vi "Abstract MVA Application (Template).vi"   [LabVIEW 2017]
uses:
  Framework/IModel/IModel/IModel.lvclass
  Framework/IViewable/IViewable/IViewable.lvclass
  Framework/IViewModel/IViewModel/IViewModel.lvclass
  C:/Git/mva-framework/Source/Framework/IViewManager/IViewManager/IViewManager.lvclass
  C:/Program Files (x86)/National Instruments/LabVIEW 2017/vi.lib/ActorFramework/Actor/Actor.lvclass
  Framework/Mediator/Mediator/Mediator.lvclass
  C:/Git/mva-framework/Source/Framework/IMediator/IMediator/IMediator.lvclass
  Framework/Mediator/MediatorBusMonitor/MediatorBusMonitor.lvclass
  C:/Git/mva-framework/Source/Framework/IMediator/IMediatorBusMonitor/MediatorBusMonitor/IMediatorBusMonitor.lvclass
  <vilib>/ActorFramework/Message Enqueuer/Message Priority.ctl
  Framework/IViewable/IViewable/View Position Enum.ctl
  Framework/IMediator/IMediator/IMediator.lvclass/IMediator.ctl
  Framework/IViewModel/IViewModel/IViewModel.lvclass/IViewModel.ctl
  Framework/IViewManager/IViewManager Messages/Launch Nested Views Msg/Launch Nested Views Msg.lvclass/Launch Nested Views Msg.ctl
  Framework/IViewManager/IViewManager/IViewManager.lvclass/IViewManager.ctl
  Framework/IViewable/IViewable Messages/Open Front Panel Msg/Open Front Panel Msg.lvclass/Open Front Panel Msg.ctl
  <vilib>/ActorFramework/Message Enqueuer/Message Enqueuer.lvclass/Message Enqueuer.ctl
  5c4f144a-bf04-4631-b5b9-56dc2cdea438.vi
  5c4f144a-bf04-4631-b5b9-56dc2cdea438.vi/e2f200b5-ebbe-407f-9208-31fbff5dbac3.vi
  Framework/IViewModel/IViewModel/Write Startup Model-View Configuration.vi
  <vilib>/ActorFramework/Message Enqueuer/Enqueue.vi
  5c4f144a-bf04-4631-b5b9-56dc2cdea438.vi/e2f200b5-ebbe-407f-9208-31fbff5dbac3.vi/ce21ce61-61c6-4c77-86d8-c0f4c29ff366.vi
  Framework/IViewManager/IViewManager Messages/Launch Nested Views Msg/Pack Launch Nested Views Msg.vi
  Framework/IViewManager/IViewManager/Write Startup Launch Nested Views Msg.vi
  gpm_packages/@cs/event-logger/Source/Text File Sink/Text File Sink.lvclass
  C:/Git/mva-framework/gpm_packages/@cs/event-logger/Source/Composed Log/Log Sink/Log Sink.lvclass
  Framework/IViewable/IViewable Messages/Open Front Panel Msg/Open Front Panel Msg.lvclass
  C:/Program Files (x86)/National Instruments/LabVIEW 2017/vi.lib/ActorFramework/Message/Message.lvclass
  gpm_packages/@cs/event-logger/Source/Composed Log/Application Logger/Write ErrorFormat.vi
  gpm_packages/@cs/event-logger/Source/Composed Log/Application Logger/Launch Worker Loop.vi
  gpm_packages/@cs/event-logger/Source/Composed Log/LoggerReference/Construct Log Instance.vi
  gpm_packages/@cs/event-logger/Source/Composed Log/Global Application Log/Logger Queue FGV.vi
  gpm_packages/@cs/event-logger/Source/Composed Log/Global Application Log/Add Single Sink.vi
  <vilib>/ActorFramework/Message Priority Queue/Priority Enqueue.vi
  gpm_packages/@cs/event-logger/Source/Composed Log/IErrorFormat/IErrorFormat.lvclass
  gpm_packages/@cs/event-logger/Source/Composed Log/Application Logger/Application Logger.lvclass
  gpm_packages/@cs/event-logger/Source/Composed Log/LoggerReference/LoggerReference.lvclass
  gpm_packages/@cs/event-logger/Source/Composed Log/Log Sink/Log Sink.lvclass
  Framework/IViewable/IApplicationStyle/IApplicationStyle.lvclass
  Framework/IViewManager/IViewManager Messages/Launch Nested Views Msg/Launch Nested Views Msg.lvclass
  <vilib>/ActorFramework/Actor/Actor.lvclass
  Framework/IMediator/IMediator/IMediator.lvclass
  <vilib>/ActorFramework/Message Enqueuer/Message Enqueuer.lvclass
  EventSinkConfigurations/EventSinkConfigurations.lvlib
panel:
  # "This example launches a simple abstract MVA application.\nReplace IModel with your Root Model or dependency-injected Model hierarchy.\nReplace IViewable with your Viewable or nested hierarchy of Viewables and ViewManagers\nReplace IViewModel with your concrete ViewModel that requests Model activity driven by user inputs\nMediator is already concrete--only replace it if you write your own Mediator"
types:
  T1 = typedef "IViewable.lvlib/IViewable.lvclass/View Position Enum.ctl" = enum16{"Centered", "Maximized", "Minimized", "Custom", "Unchanged"}
  T2 = typedef "Actor Framework.lvlib/Message Enqueuer.lvclass/Message Priority.ctl" = enum16{"Low", "Normal", "High"}
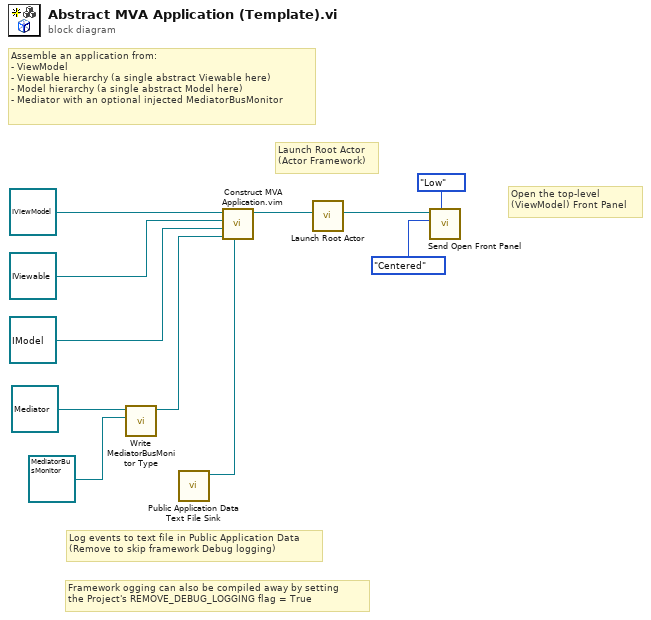
[diagram p0: block diagram]
diagram:
  # "Framework ogging can also be compiled away by setting\nthe Project's REMOVE_DEBUG_LOGGING flag = True"
  # "Log events to text file in Public Application Data\n(Remove to skip framework Debug logging)"
  # "Open the top-level\n(ViewModel) Front Panel"
  # "Launch Root Actor\n(Actor Framework)"
  # "Assemble an application from:\n- ViewModel\n- Viewable hierarchy (a single abstract Viewable here)\n- Model hierarchy (a single abstract Model here)\n- Mediator with an optional injected MediatorBusMonitor"
  n1 = call "Write MediatorBusMonitor Type.vi"("MediatorBusMonitor (Type)"=refnum<class "MediatorBusMonitor.lvclass"> refnum ("Mediator.lvlib:MediatorBusMonitor.lvclass"), "IMediator in"=refnum<class "Mediator.lvclass"> refnum ("Mediator.lvlib:Mediator.lvclass")) -> ("IMediator out"=w6:refnum<class "Mediator.lvclass">)  [unwired: 9 in]
  n2 = call "Public Application Data Text File Sink.vi"() -> ("Text File Sink"=w1:refnum<class "Text File Sink.lvclass">)  [unwired: 11 in]
  n3 = call "Construct MVA Application.vim"("Event Log Sink(s) or Sink Reference(s)"=w1, "Mediator Type"=w6, "Model Type"=refnum<class "IModel.lvclass"> refnum ("IModel.lvlib:IModel.lvclass"), "Startup View Configuration"=refnum<class "IViewable.lvclass"> refnum ("IViewable.lvlib:IViewable.lvclass"), "IViewModel In"=refnum<class "IViewModel.lvclass"> refnum ("IViewModel.lvlib:IViewModel.lvclass")) -> ("IViewModel Out"=w5:refnum<class "IViewModel.lvclass">)  [unwired: 6 in]
  n4 = call <vilib>:"Launch Root Actor.vi"("Actor"=w5) -> ("Actor's Enqueuer"=w4:refnum<class "Message Enqueuer.lvclass">)  [unwired: 9 in, 1 out]
  n5 = call "Send Open Front Panel.vi"("Message Priority (Normal)"=Message_Priority."Low", "Position"=View_Position_Enum."Centered", "Message Enqueuer"=w4) -> ()  [unwired: 7 in, 2 out]
